vi "test_CCDSetAndGetXAxisConversionType.vi"(7 "Test should pass":bool=TRUE, 8 "error in":errorcluster, 9 "tear down connection":bool=TRUE, 10 "set-up a connection":bool=TRUE, 11 "device selection":enum16{"monochromator", "CCD", "SCD"}(ring)=enum."CCD") -> (0 "error out":errorcluster)   [LabVIEW 2023]
uses:
  Source/Classes/Mono/Monochromator.lvclass
  Source/Classes/CCD/CCD.lvclass
  Source/Classes/SCD/SCD.lvclass
  <vilib>/addons/_JKI Toolkits/Caraya/classes/Assert/Assert Equal Value and Type_Variant.vi
  <vilib>/addons/_JKI Toolkits/Caraya/classes/Assert/Assert Not Error.vi
  Source/Classes/GenericDevice/GenericDevice.lvclass
  <vilib>/addons/_JKI Toolkits/Caraya/classes/Test/Test.lvclass
  <vilib>/addons/_JKI Toolkits/Caraya/classes/Assert/Assert.lvclass
  Source/Classes/CCD/XAxisConversionTypeEnum.ctl
panel:
  # "Connector Pane"
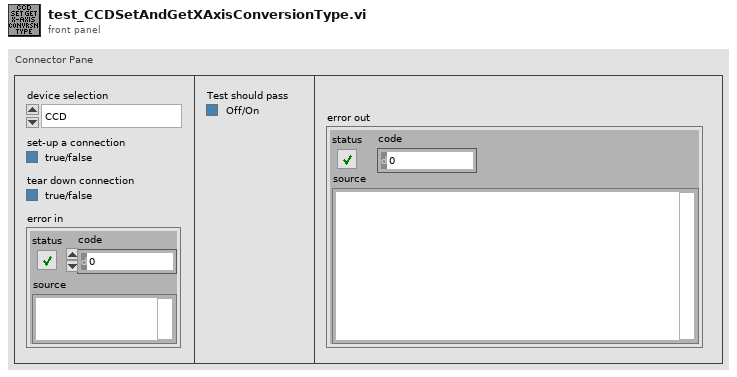
[diagram p1: front panel]
types:
  T1 = typedef "CCD.lvclass/XAxisConversionTypeEnum.ctl" = enum16{"None (default)", "CCD FIT parameters contained in the CCD firmware", "Mono Wavelength parameters contained in the icl_settings.ini file"}
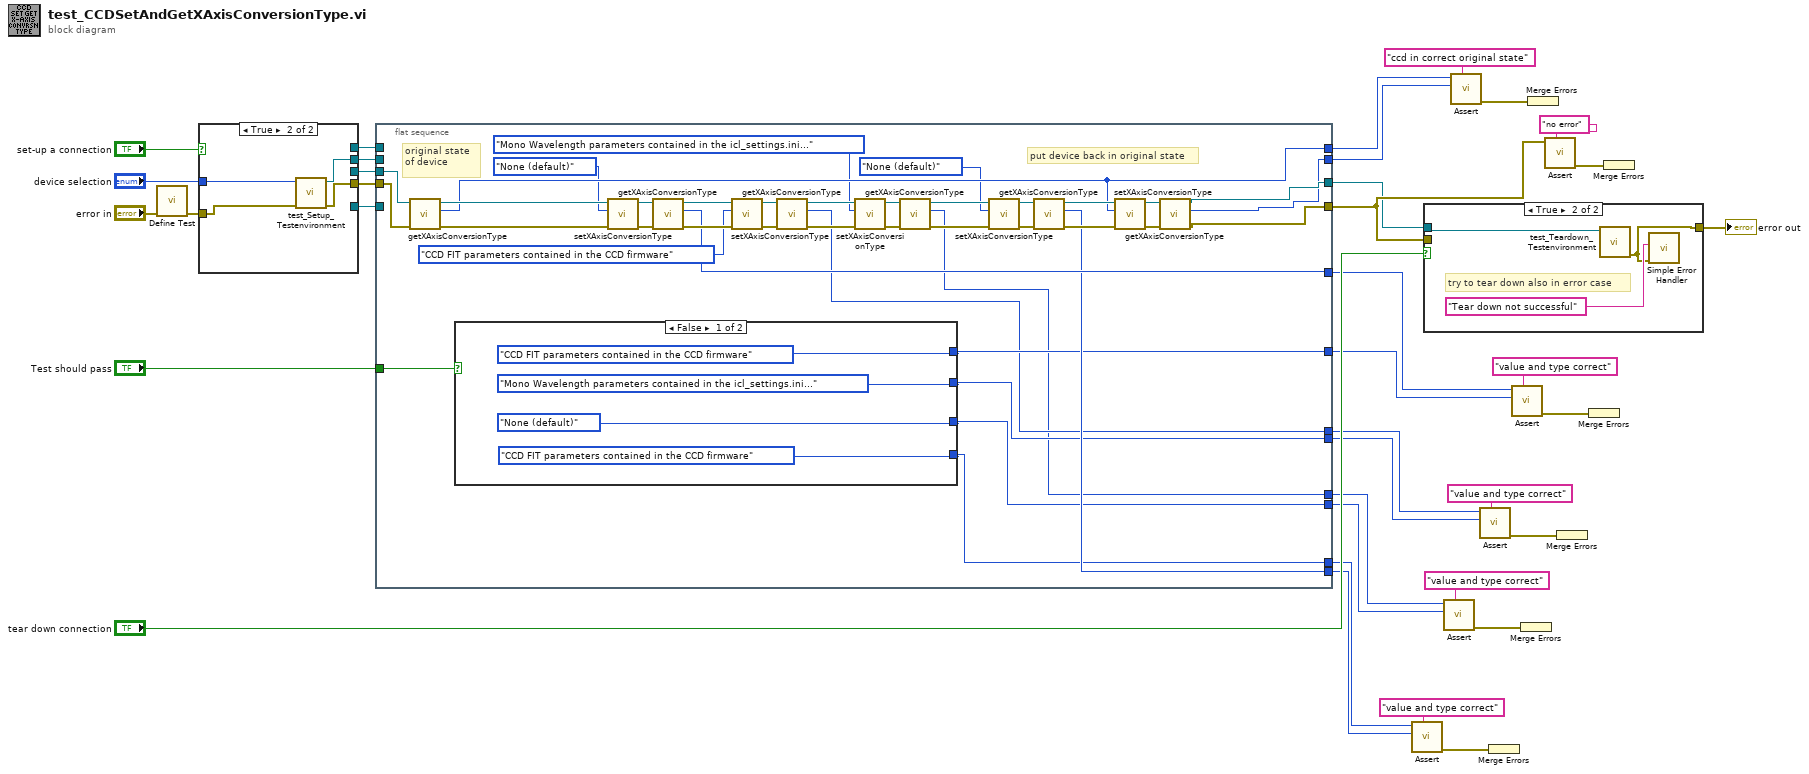
[diagram p0: block diagram]
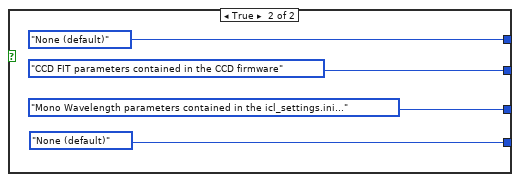
[diagram p2: hidden frame]
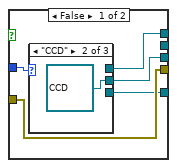
[diagram p3: hidden frame]
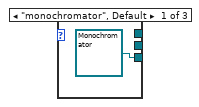
[diagram p4: hidden frame]
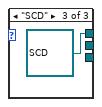
[diagram p5: hidden frame]
diagram:
  n1 = call <vilib>:"Define Test.vi"("error in (no error)"="error in") -> ("error out"=w30:errorcluster)  [unwired: 9 in, 1 out]
  n2 = case shown="True" "set-up a connection" {
    tunnel: w30 -> [w41 w48]
    tunnel: [w41 w47] -> w32
    tunnel: "device selection" -> [w40 w46]
    tunnel: [_ w45] -> w29
    tunnel: [w39 _] -> w28
    tunnel: [w38 _] -> w27
    tunnel: [w37 _] -> w26
    frame False {
      n3 = case shown="\"CCD\"" w40 {
        tunnel: [refnum<class "Monochromator.lvclass"> refnum ("Monochromator.lvclass") _ _] -> w39
        tunnel: [_ refnum<class "CCD.lvclass"> refnum ("CCD in") _] -> w38
        tunnel: [_ _ refnum<class "SCD.lvclass"> refnum ("SCD.lvclass")] -> w37
        frame "monochromator", Default {
        }
        frame "CCD" {
        }
        frame "SCD" {
        }
      }
    }
    frame True {
      n4 = call "test_Setup_Testenvironment.vi"("error in"=w48, "device selection"=w46) -> ("error out"=w47:errorcluster, "GenericDevice.lvclass"=w45:refnum<class "GenericDevice.lvclass">)  [unwired: 7 in, 1 out]
    }
  }
  n5 = flat-sequence {
    tunnel: w32 -> [w85]
    tunnel: w29 -> [_]
    tunnel: w28 -> [_]
    tunnel: w27 -> [w86]
    tunnel: w26 -> [_]
    tunnel: [w63] -> w21
    tunnel: "Test should pass" -> [w87]
    tunnel: [w62] -> w20
    tunnel: [w61] -> w17
    tunnel: [w64] -> w16
    tunnel: [w60] -> w15
    tunnel: [w57] -> w13
    tunnel: [w53] -> w11
    tunnel: [w59] -> w8
    tunnel: [w58] -> w14
    tunnel: [w56] -> w12
    tunnel: [w54] -> w10
    tunnel: [w55] -> w9
    frame #0 {
      # "put device back in original state"
      # "original state of device"
      n6 = call "getXAxisConversionType.vi"("error in (no error)"=w85, "CCD in"=w86) -> ("error out"=w65:errorcluster, "x axis conversion type"=w64:T1, "CCD out"=w66:refnum<class "CCD.lvclass">)  [unwired: 7 in]
      n7 = case shown="False" w87 {
        tunnel: [XAxisConversionTypeEnum."CCD FIT parameters contained in the CCD firmware" ("type") XAxisConversionTypeEnum."None (default)" ("type")] -> w58
        tunnel: [XAxisConversionTypeEnum."Mono Wavelength parameters contained in the icl_settings.ini file" ("type") XAxisConversionTypeEnum."CCD FIT parameters contained in the CCD firmware" ("type")] -> w56
        tunnel: [XAxisConversionTypeEnum."None (default)" ("type") XAxisConversionTypeEnum."Mono Wavelength parameters contained in the icl_settings.ini file" ("type")] -> w54
        tunnel: [XAxisConversionTypeEnum."CCD FIT parameters contained in the CCD firmware" ("type") XAxisConversionTypeEnum."None (default)" ("type")] -> w55
        frame False {
        }
        frame True {
        }
      }
      n8 = call "setXAxisConversionType.vi"("error in (no error)"=w65, "Enum"=XAxisConversionTypeEnum."None (default)" ("type"), "CCD in"=w66) -> ("error out"=w74:errorcluster, "CCD out"=w73:refnum<class "CCD.lvclass">)  [unwired: 5 in, 2 out]
      n9 = call "getXAxisConversionType.vi"("error in (no error)"=w74, "CCD in"=w73) -> ("error out"=w78:errorcluster, "x axis conversion type"=w60:T1, "CCD out"=w77:refnum<class "CCD.lvclass">)  [unwired: 7 in]
      n10 = call "setXAxisConversionType.vi"("error in (no error)"=w78, "Enum"=XAxisConversionTypeEnum."CCD FIT parameters contained in the CCD firmware" ("type"), "CCD in"=w77) -> ("error out"=w75:errorcluster, "CCD out"=w76:refnum<class "CCD.lvclass">)  [unwired: 5 in, 2 out]
      n11 = call "getXAxisConversionType.vi"("error in (no error)"=w75, "CCD in"=w76) -> ("error out"=w80:errorcluster, "x axis conversion type"=w57:T1, "CCD out"=w79:refnum<class "CCD.lvclass">)  [unwired: 7 in]
      n12 = call "setXAxisConversionType.vi"("error in (no error)"=w80, "Enum"=XAxisConversionTypeEnum."Mono Wavelength parameters contained in the icl_settings.ini file" ("type"), "CCD in"=w79) -> ("error out"=w68:errorcluster, "CCD out"=w67:refnum<class "CCD.lvclass">)  [unwired: 5 in, 2 out]
      n13 = call "getXAxisConversionType.vi"("error in (no error)"=w68, "CCD in"=w67) -> ("error out"=w72:errorcluster, "x axis conversion type"=w53:T1, "CCD out"=w71:refnum<class "CCD.lvclass">)  [unwired: 7 in]
      n14 = call "setXAxisConversionType.vi"("error in (no error)"=w72, "Enum"=XAxisConversionTypeEnum."None (default)" ("type"), "CCD in"=w71) -> ("error out"=w69:errorcluster, "CCD out"=w70:refnum<class "CCD.lvclass">)  [unwired: 5 in, 2 out]
      n15 = call "getXAxisConversionType.vi"("error in (no error)"=w69, "CCD in"=w70) -> ("error out"=w84:errorcluster, "x axis conversion type"=w59:T1, "CCD out"=w83:refnum<class "CCD.lvclass">)  [unwired: 7 in]
      n16 = call "setXAxisConversionType.vi"("error in (no error)"=w84, "Enum"=w64, "CCD in"=w83) -> ("error out"=w81:errorcluster, "CCD out"=w82:refnum<class "CCD.lvclass">)  [unwired: 5 in, 2 out]
      n17 = call "getXAxisConversionType.vi"("error in (no error)"=w81, "CCD in"=w82) -> ("error out"=w63:errorcluster, "x axis conversion type"=w61:T1, "CCD out"=w62:refnum<class "CCD.lvclass">)  [unwired: 7 in]
    }
  }
  n18 = call-poly <vilib>:"Assert.vi"("Label"="value and type correct" ("Label (VI Title)"), "Y"=w8, "X"=w9) -> ("error out"=w34:errorcluster)  [unwired: 7 in, 1 out]
  n19 = case shown="True" "tear down connection" {
    tunnel: w20 -> [_ w98]
    tunnel: [w96 w97] -> w1
    tunnel: w21 -> [w96 _]
    frame False {
    }
    frame True {
      # "try to tear down also in error case"
      n20 = call "test_Teardown_Testenvironment.vi"("GenericDevice.lvclass"=w98) -> ("error out"=w97:errorcluster)  [unwired: 9 in, 1 out]
      n21 = call <vilib>:"Simple Error Handler.vi"("error source (\" \")"="Tear down not successful" ("error source (\" \")"), "error in (no error)"=w97) -> ()  [unwired: 3 in, 5 out]
    }
  }
  "error out" <- w1
  n22 = call-poly <vilib>:"Assert.vi"("Label"="value and type correct" ("Label (VI Title)"), "Y"=w10, "X"=w11) -> ("error out"=w7:errorcluster)  [unwired: 7 in, 1 out]
  n23 = call-poly <vilib>:"Assert.vi"("Label"="ccd in correct original state" ("Label (VI Title)"), "Y"=w17, "X"=w16) -> ("error out"=w19:errorcluster)  [unwired: 7 in, 1 out]
  n24 = call-poly <vilib>:"Assert.vi"("Label"="value and type correct" ("Label (VI Title)"), "Y"=w12, "X"=w13) -> ("error out"=w3:errorcluster)  [unwired: 7 in, 1 out]
  n25 = Merge Errors(w34) -> ()  [unwired: 1 out]
  n26 = call-poly <vilib>:"Assert.vi"("Label"="value and type correct" ("Label (VI Title)"), "Y"=w14, "X"=w15) -> ("error out"=w4:errorcluster)  [unwired: 7 in, 1 out]
  n27 = Merge Errors(w7) -> ()  [unwired: 1 out]
  n28 = Merge Errors(w19) -> ()  [unwired: 1 out]
  n29 = call-poly <vilib>:"Assert.vi"("Label"="no error" ("Label (VI Title)"), "Not Error?"=w21) -> ("error out"=w23:errorcluster)  [unwired: 8 in, 1 out]
  n30 = Merge Errors(w3) -> ()  [unwired: 1 out]
  n31 = Merge Errors(w4) -> ()  [unwired: 1 out]
  n32 = Merge Errors(w23) -> ()  [unwired: 1 out]
